vi "weryfikator_peselu.vi"() -> ()   [LabVIEW 2023]
panel:
  out "DANE PO WERYFIKACJI":T1
  in  "WPROWADZ DANE DO WERYFIKACJI":T2 caption="Wprowadz dane do weryfikacji"
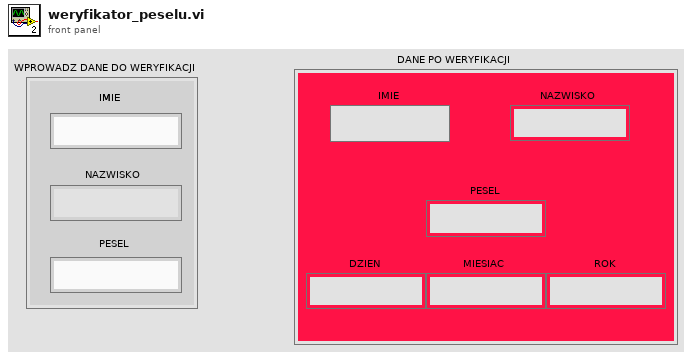
[diagram p1: front panel]
types:
  T1 = cluster{bool, "PESEL":string, "IMIE":string, "NAZWISKO":string, "ROK":string, "MIESIAC":string, "DZIEN":string}
  T2 = cluster{"IMIE":string, "NAZWISKO":string, "PESEL":string}
  T3 = cluster{bool, "PESEL":string, string, string, string, string, string}
  T4 = cluster{bool, "PESEL":string, "IMIE":string, "NAZWISKO":string, string, "PESEL":string, "PESEL":string}
  T5 = cluster{bool, "PESEL":string, "IMIE":string, "NAZWISKO":string, string, string, "PESEL":string}
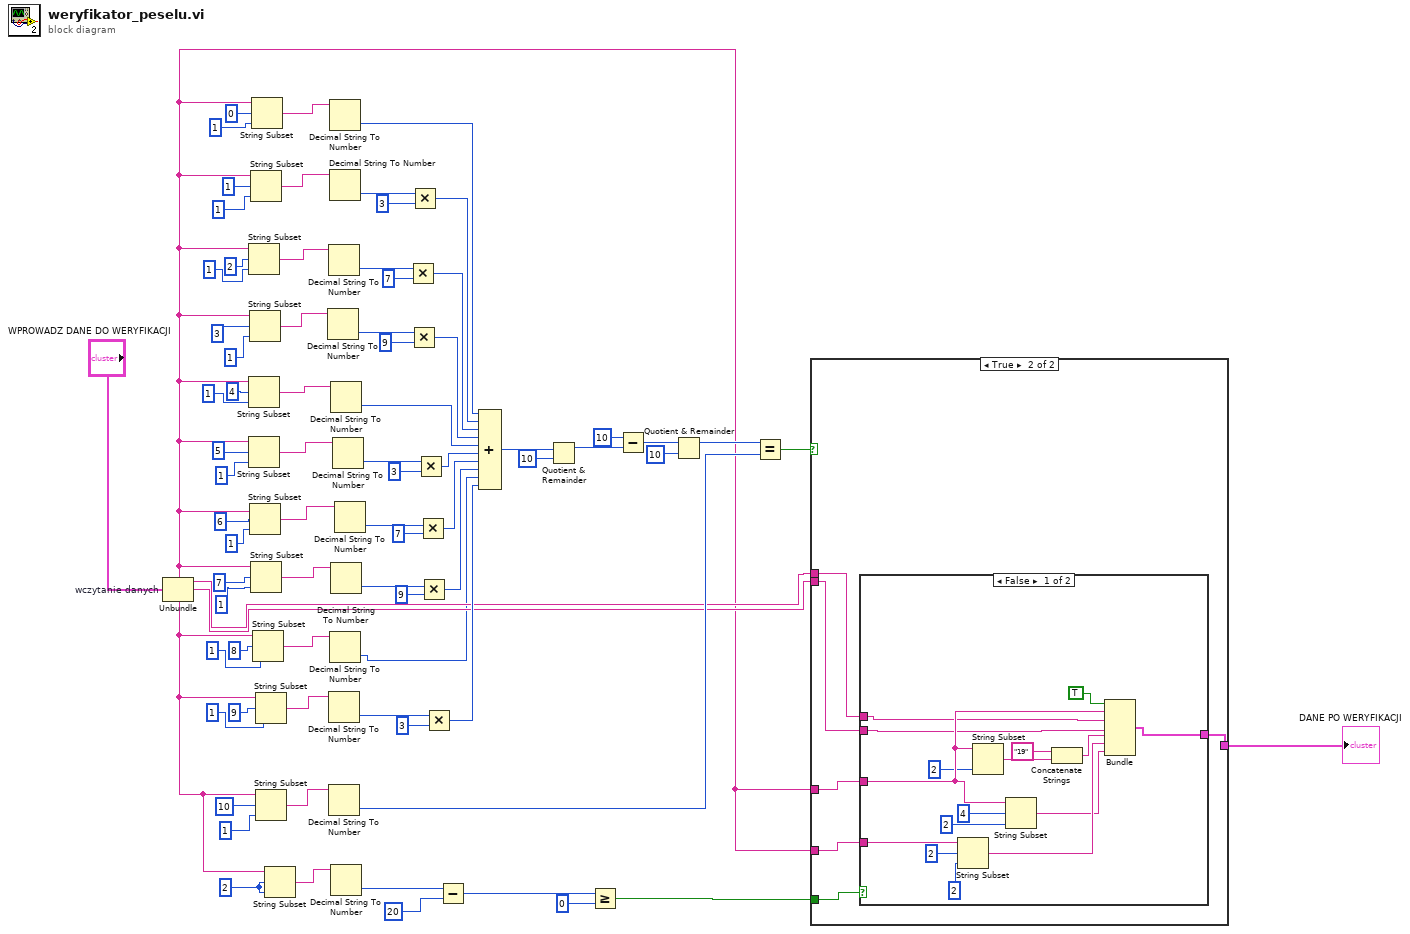
[diagram p0: block diagram]
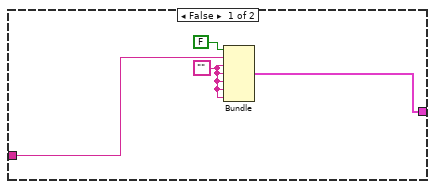
[diagram p2: hidden frame]
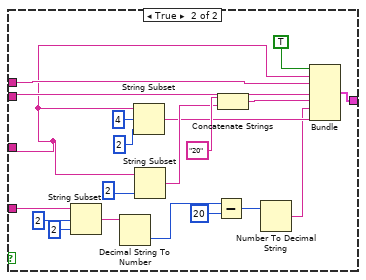
[diagram p3: hidden frame]
diagram:
  w16 = 2
  n1 = Unbundle "wczytanie danych"("WPROWADZ DANE DO WERYFIKACJI") -> ("IMIE"=w7:string, "NAZWISKO"=w8:string, "PESEL"=w5:string)
  n2 = String Subset(string=w5, offset (0)=2 ("Numeric"), length (rest)=1 ("Numeric")) -> (substring=w39:string)
  n3 = String Subset(string=w5, offset (0)=4 ("Numeric"), length (rest)=1 ("Numeric")) -> (substring=w54:string)
  n4 = String Subset(string=w5, offset (0)=5 ("Numeric"), length (rest)=1 ("Numeric")) -> (substring=w62:string)
  n5 = String Subset(string=w5, offset (0)=3 ("Numeric"), length (rest)=1 ("Numeric")) -> (substring=w47:string)
  n6 = String Subset(string=w5, offset (0)=6 ("Numeric"), length (rest)=1 ("Numeric")) -> (substring=w61:string)
  n7 = String Subset(string=w5, offset (0)=1 ("Numeric"), length (rest)=1 ("Numeric")) -> (substring=w35:string)
  n8 = String Subset(string=w5, offset (0)=7 ("Numeric"), length (rest)=1 ("Numeric")) -> (substring=w69:string)
  n9 = String Subset(string=w5, offset (0)=0 ("Numeric"), length (rest)=1 ("Numeric")) -> (substring=w28:string)
  n10 = String Subset(string=w5, offset (0)=8 ("Numeric"), length (rest)=1 ("Numeric")) -> (substring=w70:string)
  n11 = String Subset(string=w5, offset (0)=9 ("Numeric"), length (rest)=1 ("Numeric")) -> (substring=w75:string)
  n12 = String Subset(string=w5, offset (0)=10 ("Numeric"), length (rest)=1 ("Numeric")) -> (substring=w19:string)
  n13 = String Subset(string=w5, offset (0)=w16, length (rest)=w16) -> (substring=w15:string)
  n14 = Decimal String To Number(string=w47) -> (number=w44:i32)  [unwired: 2 in, 1 out]
  n15 = Decimal String To Number(string=w39) -> (number=w38:i32)  [unwired: 2 in, 1 out]
  n16 = Decimal String To Number(string=w75) -> (number=w74:i32)  [unwired: 2 in, 1 out]
  n17 = Decimal String To Number(string=w19) -> (number=w17:i32)  [unwired: 2 in, 1 out]
  n18 = Decimal String To Number(string=w28) -> (number=w1:i32)  [unwired: 2 in, 1 out]
  n19 = Decimal String To Number(string=w35) -> (number=w34:i32)  [unwired: 2 in, 1 out]
  n20 = Decimal String To Number(string=w70) -> (number=w3:i32)  [unwired: 2 in, 1 out]
  n21 = Decimal String To Number(string=w54) -> (number=w2:i32)  [unwired: 2 in, 1 out]
  n22 = Decimal String To Number(string=w69) -> (number=w58:i32)  [unwired: 2 in, 1 out]
  n23 = Decimal String To Number(string=w15) -> (number=w14:i32)  [unwired: 2 in, 1 out]
  n24 = Decimal String To Number(string=w62) -> (number=w56:i32)  [unwired: 2 in, 1 out]
  n25 = Decimal String To Number(string=w61) -> (number=w57:i32)  [unwired: 2 in, 1 out]
  n26 = Multiply(x=w38, y=7 ("Numeric")) -> (x*y=w36:i32)
  n27 = Multiply(x=w44, y=9 ("Numeric")) -> (x*y=w42:i32)
  n28 = Multiply(x=w34, y=3 ("Numeric")) -> (x*y=w31:i32)
  n29 = Multiply(x=w56, y=3 ("Numeric")) -> (x*y=w48:i32)
  n30 = Multiply(x=w57, y=7 ("Numeric")) -> (x*y=w49:i32)
  n31 = Multiply(x=w58, y=9) -> (x*y=w50:i32)
  n32 = Multiply(x=w74, y=3) -> (x*y=w51:i32)
  n33 = Subtract(x=w14, y=20) -> (x-y=w12:i32)
  n34 = Compound Arithmetic op=ADD(w1, w31, w36, w42, w2, w48, w49, w50, w3, w51) -> (w27:i32)
  n35 = Quotient & Remainder(x=w27, y=10) -> (x-y*floor(x/y)=w25:i32)  [unwired: 1 out]
  n36 = Greater Or Equal?(x=w12, y=0) -> (x >= y?=w9:bool)
  n37 = Subtract(x=10, y=w25) -> (x-y=w23:i32)
  n38 = Quotient & Remainder(x=w23, y=10) -> (x-y*floor(x/y)=w18:i32)  [unwired: 1 out]
  n39 = Equal?(x=w18, y=w17) -> (x = y?=w10:bool)
  n40 = case shown="True" w10 {
    tunnel: w9 -> [_ w88]
    tunnel: w8 -> [_ w85]
    tunnel: w7 -> [_ w84]
    tunnel: w5 -> [_ w86]
    tunnel: w5 -> [w80 w87]
    tunnel: [w79 w83] -> w6
    frame False {
      w81 = ""
      n41 = Bundle(FALSE, "PESEL"=w80, w81, w81, w81, w81, w81) -> (w79:T3)  [unwired: 1 in]
    }
    frame True {
      n42 = case shown="False" w88 {
        tunnel: w87 -> [w99 w110]
        tunnel: w86 -> [w103 w111]
        tunnel: w85 -> [w91 w112]
        tunnel: w84 -> [w92 w113]
        tunnel: [w100 w109] -> w83
        frame False {
          n43 = String Subset(string=w103, offset (0)=2, length (rest)=2) -> (substring=w101:string)
          n44 = String Subset(string=w99, length (rest)=2) -> (substring=w95:string)  [unwired: 1 in]
          n45 = String Subset(string=w99, offset (0)=4, length (rest)=2) -> (substring=w98:string)
          n46 = Concatenate Strings("19", w95) -> (w93:string)
          n47 = Bundle(TRUE, "PESEL"=w99, "IMIE"=w92, "NAZWISKO"=w91, w93, "PESEL"=w101, "PESEL"=w98) -> (w100:T4)  [unwired: 1 in]
        }
        frame True {
          n48 = String Subset(string=w111, offset (0)=2, length (rest)=2) -> (substring=w118:string)
          n49 = Decimal String To Number(string=w118) -> (number=w117:i32)  [unwired: 2 in, 1 out]
          n50 = String Subset(string=w110, offset (0)=4, length (rest)=2) -> (substring=w119:string)
          n51 = String Subset(string=w110, length (rest)=2) -> (substring=w122:string)  [unwired: 1 in]
          n52 = Subtract(x=w117, y=20) -> (x-y=w115:i32)
          n53 = Concatenate Strings("20", w122) -> (w121:string)
          n54 = Number To Decimal String(number=w115) -> (decimal integer string=w114:string)  [unwired: 1 in]
          n55 = Bundle(TRUE, "PESEL"=w110, "IMIE"=w113, "NAZWISKO"=w112, w121, w114, "PESEL"=w119) -> (w109:T5)  [unwired: 1 in]
        }
      }
    }
  }
  "DANE PO WERYFIKACJI" <- w6
